vi "LVClass_HasoEngine Write HasoEngine.vi"(8 "error in (no error)":errorcluster, 10 "HasoEngine":T1, 11 "HasoEngine in":refnum<class "HasoEngine.lvclass">) -> (0 "error out":errorcluster, 3 "HasoEngine out":refnum<class "HasoEngine.lvclass">)   [LabVIEW 2020, in "HasoEngine.lvclass"]
uses:
  HasoEngine.lvclass
  ClassID.ctl
  Handle creation.ctl
  HasoEngine.lvclass/HasoEngine.ctl
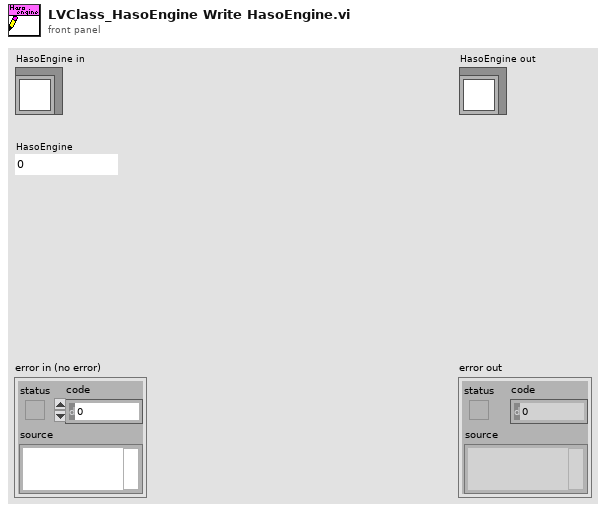
[diagram p1: front panel]
types:
  T1 = typedef "ClassID.ctl" = i64
  T2 = typedef "Handle creation.ctl" = enum16{"By ctor", "By write function"}
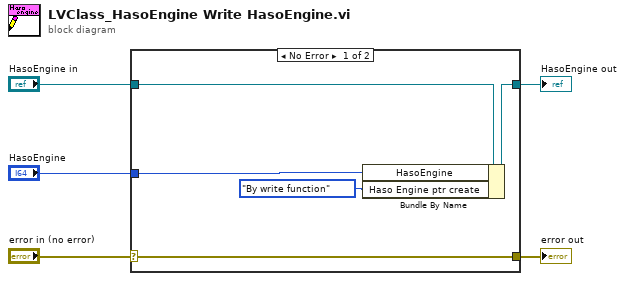
[diagram p0: block diagram]
diagram:
  n1 = case shown="No Error" "error in (no error)" {
    selector: "error in (no error)" -> [w10 w11]
    tunnel: [w10 w11] -> w4
    tunnel: [w8 w12] -> w2
    tunnel: "HasoEngine in" -> [w9 w12]
    tunnel: "HasoEngine" -> [w7 _]
    frame No Error {
      n2 = Bundle By Name(cluster=w9, "HasoEngine"=w7, "Haso Engine ptr create"=Handle_creation."By write function") -> (w8:refnum<class "HasoEngine.lvclass">)
    }
    frame Error {
    }
  }
  "error out" <- w4
  "HasoEngine out" <- w2
